vi "Calc Hight of Camera in inches.vi"(0 "Target":T1, 1 "width of T in inches":i32=21) -> (8 "Width in inches":dbl)   [LabVIEW 2016]
panel:
  in  "width C in pixels":i32=240
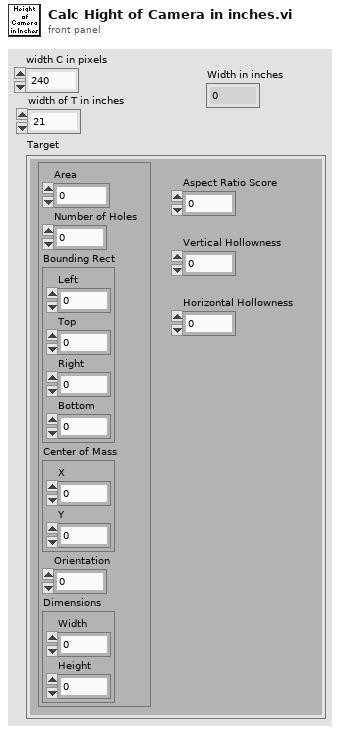
[diagram p1: front panel]
types:
  T1 = cluster{"Particle Report":cluster{"Area":dbl, "Number of Holes":dbl, "Bounding Rect":cluster{"Left":dbl, "Top":dbl, "Right":dbl, "Bottom":dbl}, "Center of Mass":cluster{"X":dbl, "Y":dbl}, "Orientation":dbl, "Dimensions":cluster{"Width":dbl, "Height":dbl}}, "Aspect Ratio Score":dbl, "Vertical Hollowness":dbl, "Horizontal Hollowness":dbl}
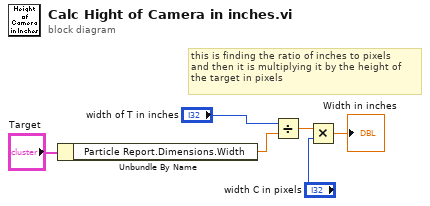
[diagram p0: block diagram]
diagram:
  # "this is finding the ratio of inches to pixels \nand then it is multiplying it by the height of\nthe target in pixels"
  n1 = Unbundle By Name("Target") -> ("Particle Report.Dimensions.Width"=w5:dbl)
  n2 = Divide(x="width of T in inches", y=w5) -> (x/y=w3:dbl)
  n3 = Multiply(x=w3, y="width C in pixels") -> (x*y=→"Width in inches":dbl)
